vi "UpdateData.vi"(6 "Delay Time":sgl[](array[numeric]), 7 "Detector Select":enum32{"4 Detectors", "8 Detectors"}(radio)=enum."8 Detectors", 8 "Duration Time (ms)":sgl) -> (0 "g2 data":string, 1 "tau data":string, 2 "Intensity data":string, 3 "g2 Display":cluster{"Delay Time":sgl[], sgl[]}[](array[cluster]), 4 "Tau Array":sgl[](array[numeric]), 5 "Intensity Array":sgl[](array[numeric]), 9 "Elapsed Time(s)":sgl)   [LabVIEW 2011]
uses:
  flex05oem8chautoPASCAL.dll
  flex05-4chPascal.dll
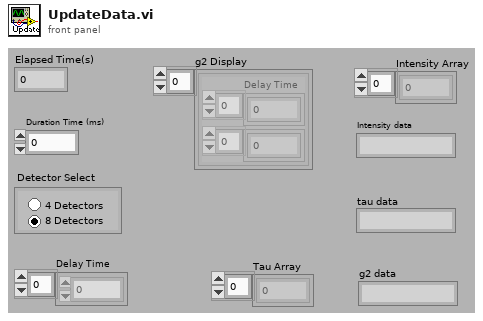
[diagram p1: front panel]
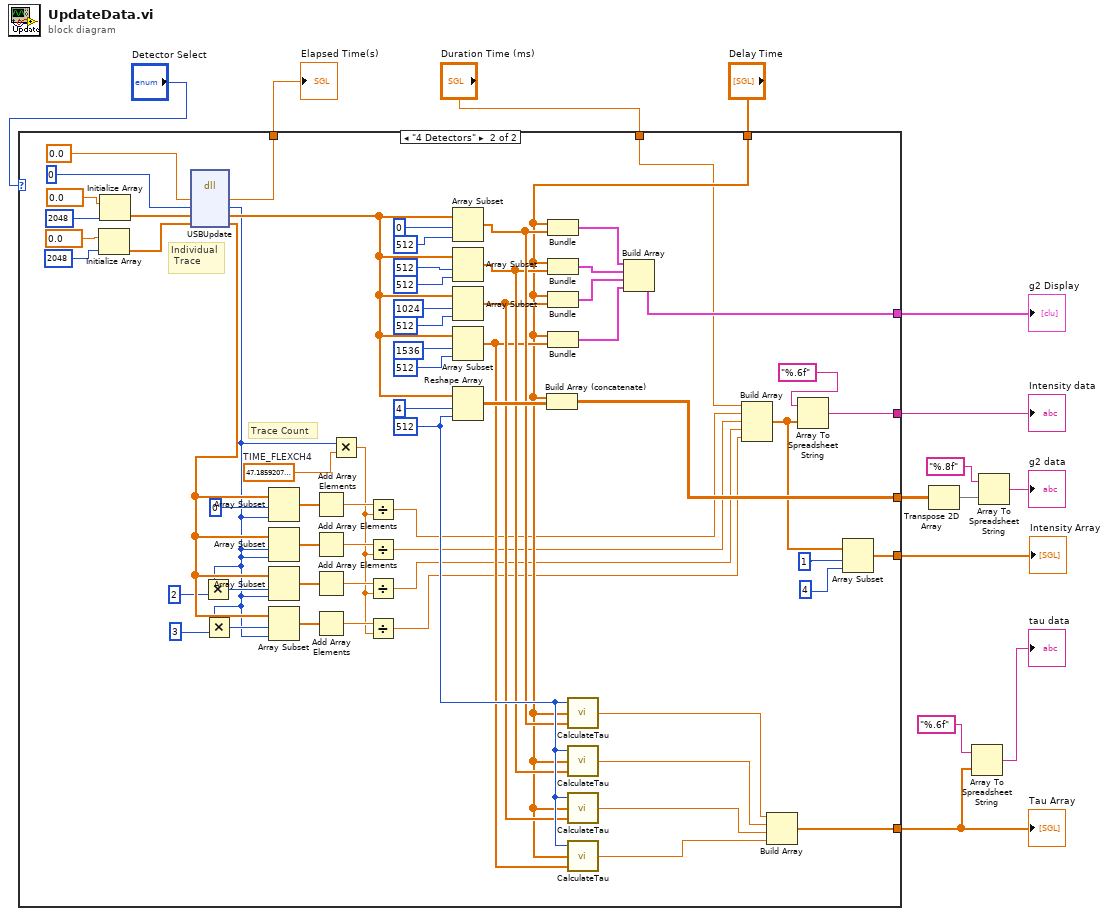
[diagram p0: block diagram]
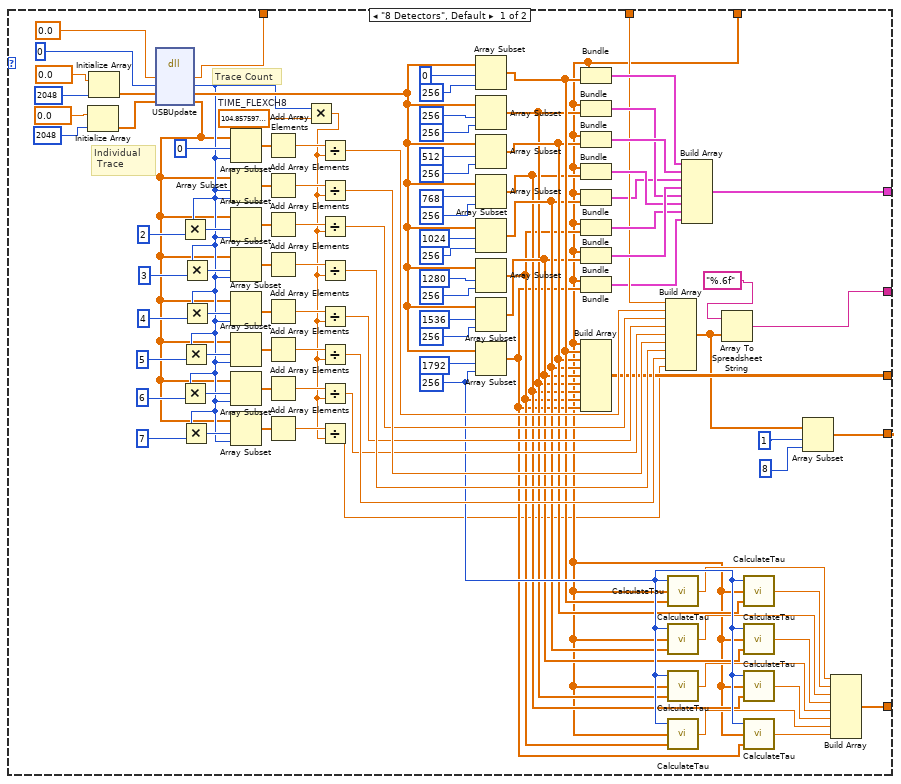
[diagram p2: hidden frame]
diagram:
  n1 = case shown="\"4 Detectors\"" "Detector Select" {
    tunnel: [w32 w168] -> w9
    tunnel: [w100 w167] -> w11
    tunnel: [w50 w165] -> w4
    tunnel: "Duration Time (ms)" -> [w61 w117]
    tunnel: [w53 w146] -> w10
    tunnel: "Delay Time" -> [w30 w136]
    tunnel: [w29 w135] -> w7
    tunnel: [w25 w119] -> w14
    frame "8 Detectors", Default {
      w90 = sgl 104.8576  # TIME_FLEXCH8
      w49 = 256
      # "Individual\n Trace"
      # "Trace Count"
      n2 = Initialize Array(sgl 0.0 ("Element Data"), 2048 ("Dimension Size")) -> (w18:sgl[])
      n3 = Initialize Array(sgl 0.0 ("Element Data"), 2048 ("Dimension Size")) -> (w19:sgl[])
      n4 = dll-call lib="C:/LABVIEWcodesWorksInC/UnderDeveopmentNeedChecking/Vincent2017/Dependencies/DCS/flex05oem8chautoPASCAL.dll" fn="USBUpdate" label="UpdateCH8"("arg1"=sgl 0.0 ("Input Value"), "arg2"=u16 0 ("Input Value"), "arg3"=w19, "arg4"=w18) -> ("arg1"=w32:sgl, "arg2"=w62:u16, "arg3"=w80:sgl[], "arg4"=w31:sgl[])  [unwired: 4 in, 2 out]
      n5 = Multiply(x=w62, y=2) -> (x*y=w74:i32)
      n6 = Multiply(x=w62, y=6) -> (x*y=w71:i32)
      n7 = Multiply(x=w62, y=5) -> (x*y=w72:i32)
      n8 = Multiply(x=w62, y=7) -> (x*y=w70:i32)
      n9 = Multiply(x=w62, y=3) -> (x*y=w69:i32)
      n10 = Multiply(x=w62, y=4) -> (x*y=w73:i32)
      n11 = Array Subset(array=w31, index=0, length=w62) -> (w98:sgl[])
      n12 = Array Subset(array=w31, index=w62, length=w62) -> (w97:sgl[])
      n13 = Array Subset(array=w31, index=w74, length=w62) -> (w96:sgl[])
      n14 = Array Subset(array=w31, index=w69, length=w62) -> (w95:sgl[])
      n15 = Array Subset(array=w31, index=w73, length=w62) -> (w94:sgl[])
      n16 = Array Subset(array=w31, index=w72, length=w62) -> (w93:sgl[])
      n17 = Array Subset(array=w31, index=w71, length=w62) -> (w92:sgl[])
      n18 = Array Subset(array=w31, index=w70, length=w62) -> (w91:sgl[])
      n19 = Add Array Elements(numeric array=w98) -> (sum=w89:sgl)
      n20 = Add Array Elements(numeric array=w97) -> (sum=w88:sgl)
      n21 = Add Array Elements(numeric array=w96) -> (sum=w87:sgl)
      n22 = Add Array Elements(numeric array=w95) -> (sum=w86:sgl)
      n23 = Add Array Elements(numeric array=w94) -> (sum=w85:sgl)
      n24 = Add Array Elements(numeric array=w93) -> (sum=w84:sgl)
      n25 = Add Array Elements(numeric array=w92) -> (sum=w83:sgl)
      n26 = Add Array Elements(numeric array=w91) -> (sum=w82:sgl)
      n27 = Multiply(x=w62, y=w90) -> (x*y=w81:sgl)
      n28 = Divide(x=w89, y=w81) -> (x/y=w54:sgl)
      n29 = Divide(x=w88, y=w81) -> (x/y=w58:sgl)
      n30 = Divide(x=w87, y=w81) -> (x/y=w55:sgl)
      n31 = Divide(x=w86, y=w81) -> (x/y=w59:sgl)
      n32 = Divide(x=w85, y=w81) -> (x/y=w56:sgl)
      n33 = Divide(x=w84, y=w81) -> (x/y=w60:sgl)
      n34 = Divide(x=w83, y=w81) -> (x/y=w57:sgl)
      n35 = Divide(x=w82, y=w81) -> (x/y=w16:sgl)
      n36 = Array Subset(array=w80, index=0, length=256) -> (w48:sgl[])
      n37 = Array Subset(array=w80, index=256, length=256) -> (w44:sgl[])
      n38 = Array Subset(array=w80, index=512, length=256) -> (w47:sgl[])
      n39 = Array Subset(array=w80, index=768, length=256) -> (w43:sgl[])
      n40 = Array Subset(array=w80, index=1024, length=256) -> (w46:sgl[])
      n41 = Array Subset(array=w80, index=1280, length=256) -> (w42:sgl[])
      n42 = Array Subset(array=w80, index=1536, length=256) -> (w45:sgl[])
      n43 = Array Subset(array=w80, index=1792, length=w49) -> (w41:sgl[])
      n44 = Bundle("Delay Time"=w30, w48) -> (w108:cluster{"Delay Time":sgl[], sgl[]})  [unwired: 1 in]
      n45 = Bundle("Delay Time"=w30, w44) -> (w77:cluster{"Delay Time":sgl[], sgl[]})  [unwired: 1 in]
      n46 = Bundle("Delay Time"=w30, w47) -> (w79:cluster{"Delay Time":sgl[], sgl[]})  [unwired: 1 in]
      n47 = Bundle("Delay Time"=w30, w43) -> (w76:cluster{"Delay Time":sgl[], sgl[]})  [unwired: 1 in]
      n48 = Bundle("Delay Time"=w30, w46) -> (w51:cluster{"Delay Time":sgl[], sgl[]})  [unwired: 1 in]
      n49 = Bundle("Delay Time"=w30, w42) -> (w75:cluster{"Delay Time":sgl[], sgl[]})  [unwired: 1 in]
      n50 = Bundle("Delay Time"=w30, w45) -> (w78:cluster{"Delay Time":sgl[], sgl[]})  [unwired: 1 in]
      n51 = Bundle("Delay Time"=w30, w41) -> (w52:cluster{"Delay Time":sgl[], sgl[]})  [unwired: 1 in]
      n52 = Build Array(w30, w48, w47, w46, w45, w44, w43, w42, w41) -> (w50:sgl[][])
      n53 = Build Array(w61, w54, w55, w56, w57, w58, w59, w60, w16) -> (w15:sgl[])
      n54 = call "CalculateTau.vi"("g2 data"=w48, "delaytime"=w30, "array size"=w49) -> ("Tau"=w40:sgl)
      n55 = call "CalculateTau.vi"("g2 data"=w46, "delaytime"=w30, "array size"=w49) -> ("Tau"=w38:sgl)
      n56 = call "CalculateTau.vi"("g2 data"=w44, "delaytime"=w30, "array size"=w49) -> ("Tau"=w36:sgl)
      n57 = call "CalculateTau.vi"("g2 data"=w42, "delaytime"=w30, "array size"=w49) -> ("Tau"=w34:sgl)
      n58 = Build Array(w108, w79, w51, w78, w77, w76, w75, w52) -> (w100:cluster{"Delay Time":sgl[], sgl[]}[])
      n59 = Array To Spreadsheet String(array=w15, 3:"%.6f") -> (spreadsheet string=w53:string)  [unwired: 1 in]
      n60 = call "CalculateTau.vi"("g2 data"=w47, "delaytime"=w30, "array size"=w49) -> ("Tau"=w39:sgl)
      n61 = call "CalculateTau.vi"("g2 data"=w45, "delaytime"=w30, "array size"=w49) -> ("Tau"=w37:sgl)
      n62 = call "CalculateTau.vi"("g2 data"=w43, "delaytime"=w30, "array size"=w49) -> ("Tau"=w35:sgl)
      n63 = call "CalculateTau.vi"("g2 data"=w41, "delaytime"=w30, "array size"=w49) -> ("Tau"=w33:sgl)
      n64 = Array Subset(array=w15, index=1, length=8) -> (w25:sgl[])
      n65 = Build Array(w40, w39, w38, w37, w36, w35, w34, w33) -> (w29:sgl[])
    }
    frame "4 Detectors" {
      w162 = sgl 47.18592  # TIME_FLEXCH4
      w145 = 512
      # "Individual\n Trace"
      # "Trace Count"
      n66 = Initialize Array(sgl 0.0 ("Element Data"), 2048 ("Dimension Size")) -> (w122:sgl[])
      n67 = Initialize Array(sgl 0.0 ("Element Data"), 2048 ("Dimension Size")) -> (w123:sgl[])
      n68 = dll-call lib="C:/LABVIEWcodesWorksInC/UnderDeveopmentNeedChecking/Vincent2017/Dependencies/DCS/flex05-4chPascal.dll" fn="USBUpdate" label="UpdateCH4"(sgl 0.0 ("Input Value"), u16 0 ("Input Value"), w123, "arg4"=w122) -> (w168:sgl, w147:u16, w152:sgl[], "arg4"=w163:sgl[])  [unwired: 4 in, 2 out]
      n69 = Multiply(x=w147, y=2) -> (x*y=w150:i32)
      n70 = Multiply(x=w147, y=3) -> (x*y=w148:i32)
      n71 = Array Subset(array=w163, index=0, length=w147) -> (w157:sgl[])
      n72 = Array Subset(array=w163, index=w147, length=w147) -> (w156:sgl[])
      n73 = Array Subset(array=w163, index=w150, length=w147) -> (w155:sgl[])
      n74 = Array Subset(array=w163, index=w148, length=w147) -> (w154:sgl[])
      n75 = Add Array Elements(numeric array=w157) -> (sum=w161:sgl)
      n76 = Add Array Elements(numeric array=w156) -> (sum=w160:sgl)
      n77 = Add Array Elements(numeric array=w155) -> (sum=w159:sgl)
      n78 = Add Array Elements(numeric array=w154) -> (sum=w158:sgl)
      n79 = Multiply(x=w147, y=w162) -> (x*y=w153:sgl)
      n80 = Divide(x=w161, y=w153) -> (x/y=w134:sgl)
      n81 = Divide(x=w160, y=w153) -> (x/y=w133:sgl)
      n82 = Divide(x=w159, y=w153) -> (x/y=w132:sgl)
      n83 = Divide(x=w158, y=w153) -> (x/y=w131:sgl)
      n84 = Array Subset(array=w152, index=0, length=512) -> (w144:sgl[])
      n85 = Array Subset(array=w152, index=512, length=512) -> (w143:sgl[])
      n86 = Array Subset(array=w152, index=1024, length=512) -> (w142:sgl[])
      n87 = Array Subset(array=w152, index=1536, length=512) -> (w141:sgl[])
      n88 = Reshape Array(w152, 4, w145) -> (w166:sgl[][])
      n89 = Build Array (concatenate)(w136, w166) -> (w165:sgl[][])
      n90 = Bundle("Delay Time"=w136, w144) -> (w172:cluster{"Delay Time":sgl[], sgl[]})  [unwired: 1 in]
      n91 = Bundle("Delay Time"=w136, w143) -> (w171:cluster{"Delay Time":sgl[], sgl[]})  [unwired: 1 in]
      n92 = Bundle("Delay Time"=w136, w142) -> (w170:cluster{"Delay Time":sgl[], sgl[]})  [unwired: 1 in]
      n93 = Bundle("Delay Time"=w136, w141) -> (w169:cluster{"Delay Time":sgl[], sgl[]})  [unwired: 1 in]
      n94 = call "CalculateTau.vi"("g2 data"=w144, "delaytime"=w136, "array size"=w145) -> ("Tau"=w140:sgl)
      n95 = call "CalculateTau.vi"("g2 data"=w143, "delaytime"=w136, "array size"=w145) -> ("Tau"=w139:sgl)
      n96 = call "CalculateTau.vi"("g2 data"=w142, "delaytime"=w136, "array size"=w145) -> ("Tau"=w138:sgl)
      n97 = call "CalculateTau.vi"("g2 data"=w141, "delaytime"=w136, "array size"=w145) -> ("Tau"=w137:sgl)
      n98 = Build Array(w172, w171, w170, w169) -> (w167:cluster{"Delay Time":sgl[], sgl[]}[])
      n99 = Build Array(w117, w134, w133, w132, w131) -> (w118:sgl[])
      n100 = Build Array(w140, w139, w138, w137) -> (w135:sgl[])
      n101 = Array To Spreadsheet String(array=w118, 3:"%.6f") -> (spreadsheet string=w146:string)  [unwired: 1 in]
      n102 = Array Subset(array=w118, index=1, length=4) -> (w119:sgl[])
    }
  }
  "Intensity Array" <- w14
  "Tau Array" <- w7
  "g2 Display" <- w11
  "Intensity data" <- w10
  "Elapsed Time(s)" <- w9
  n103 = Transpose 2D Array(2D array=w4) -> (transposed array=w5:sgl[][])
  n104 = Array To Spreadsheet String(array=w7, 3:"%.6f") -> (spreadsheet string=→"tau data":string)  [unwired: 1 in]
  n105 = Array To Spreadsheet String(array=w5, 3:"%.8f") -> (spreadsheet string=→"g2 data":string)  [unwired: 1 in]
